vi "Read Measurement 2 Channels.vi"(8 "error in (no error)":errorcluster, 11 "Scope 2 Test in":refnum<class "Scope 2 Test.lvclass">) -> (0 "error out":errorcluster, 3 "Scope 2 Test out":refnum<class "Scope 2 Test.lvclass">)   [LabVIEW 2020, in "Oscilloscope VI.lvlib" / "Scope 2 Test.lvclass"]
uses:
  Scope 2 Test.lvclass
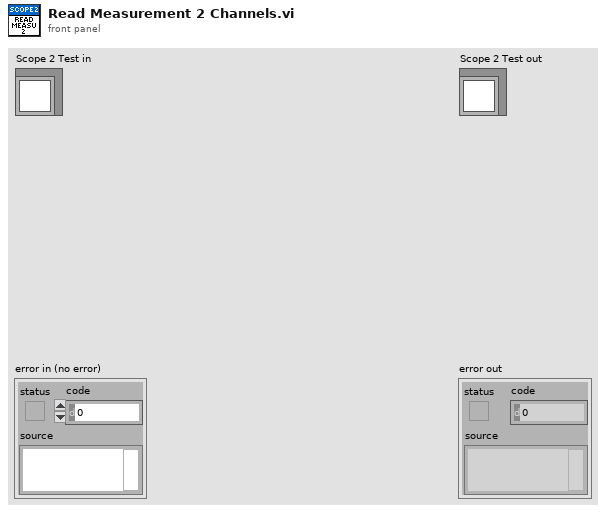
[diagram p1: front panel]
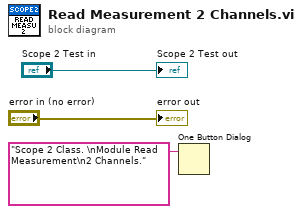
[diagram p0: block diagram]
diagram:
  n1 = One Button Dialog(message="Scope 2 Class. \nModule Read Measurement\n2 Channels.") -> ()  [unwired: 1 in, 1 out]
  "error out" <- "error in (no error)"
  "Scope 2 Test out" <- "Scope 2 Test in"
